vi "SweepCtrlSineCurrent_ver1.0.vi"(7 "Keithley 6221":T1={"Delta "=FALSE, "Const I "=FALSE, "Pulse Delta "=FALSE, "Sine Wave "=FALSE, "From I_HI (A)"=0.0, "From I (A)"=0.0, "I_LO (A)"=0.0, "From I_H (A)"=0.0, "I_L (A)"=0.0, "Freq (Hz)"=13.259, "From I_Sin (A)"=0.0, "DC Offset (A)"=0.0, "Delay Time (s)"=1.0, "Pulse Width (s)"=0.012, "Delay (s)"=0.011966, "To I (A)"=0.0, "ASymmetric?"=FALSE, "To I_HI (A)"=0.0, "To I_H (A)"=0.0, "To I_Sin (A)"=0.0, "GPIB ADR"=0, "Sweep Mode"=0, "Delta Unit"="V", "2182A range (V)"=0.01, "6221 Compliance (V)"=10.0} {"Sweep Mode" items=["Linear", "Log", "Exp", "Inverse", "Manual"]; "GPIB ADR" items=["None"=0, "12"=12, "13"=13]; "To I_Sin (A)" format="%#.5p"; "To I_H (A)" format="%#.5p"; "To I_HI (A)" format="%#.5p"; "To I (A)" format="%#.5p"; "Delay (s)" format="%.3p"; "Pulse Width (s)" format="%.3p"; "Delay Time (s)" format="%#.5p"; "DC Offset (A)" format="%#.5p"; "From I_Sin (A)" format="%#.5p"; "Freq (Hz)" format="%#_6p"; "I_L (A)" format="%#.5p"; "From I_H (A)" format="%#.5p"; "I_LO (A)" format="%#.5p"; "From I (A)" format="%#.5p"; "From I_HI (A)" format="%#.5p"}, 8 "error in (no error)":errorcluster, 9 "Set pt change flag":bool, 10 "DC St. Pt.":dbl, 11 "GPIB ADR":u16) -> (0 "error out":errorcluster)   [LabVIEW 2012]
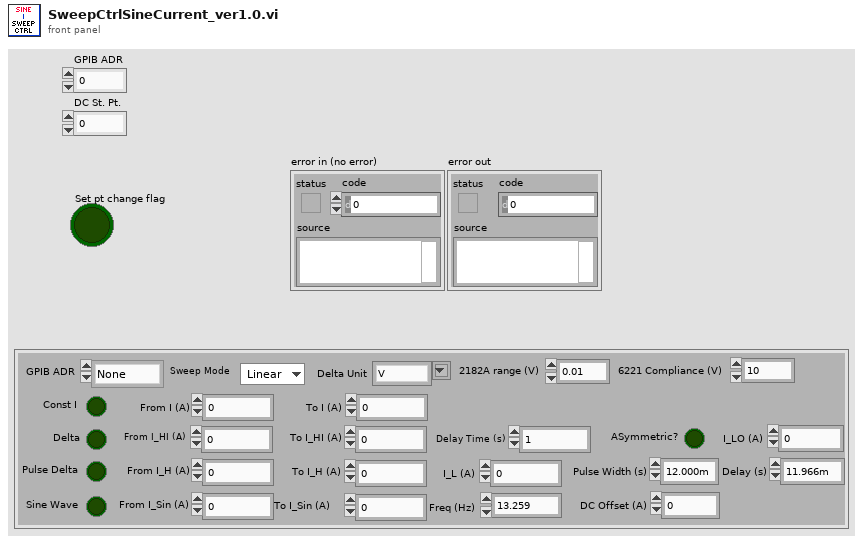
[diagram p1: front panel]
types:
  T1 = cluster{"Delta ":bool, "Const I ":bool, "Pulse Delta ":bool, "Sine Wave ":bool, "From I_HI (A)":dbl, "From I (A)":dbl, "I_LO (A)":dbl, "From I_H (A)":dbl, "I_L (A)":dbl, "Freq (Hz)":dbl, "From I_Sin (A)":dbl, "DC Offset (A)":dbl, "Delay Time (s)":dbl, "Pulse Width (s)":dbl, "Delay (s)":dbl, "To I (A)":dbl, "ASymmetric?":bool, "To I_HI (A)":dbl, "To I_H (A)":dbl, "To I_Sin (A)":dbl, "GPIB ADR":u16, "Sweep Mode":u8, "Delta Unit":string, "2182A range (V)":dbl, "6221 Compliance (V)":dbl}
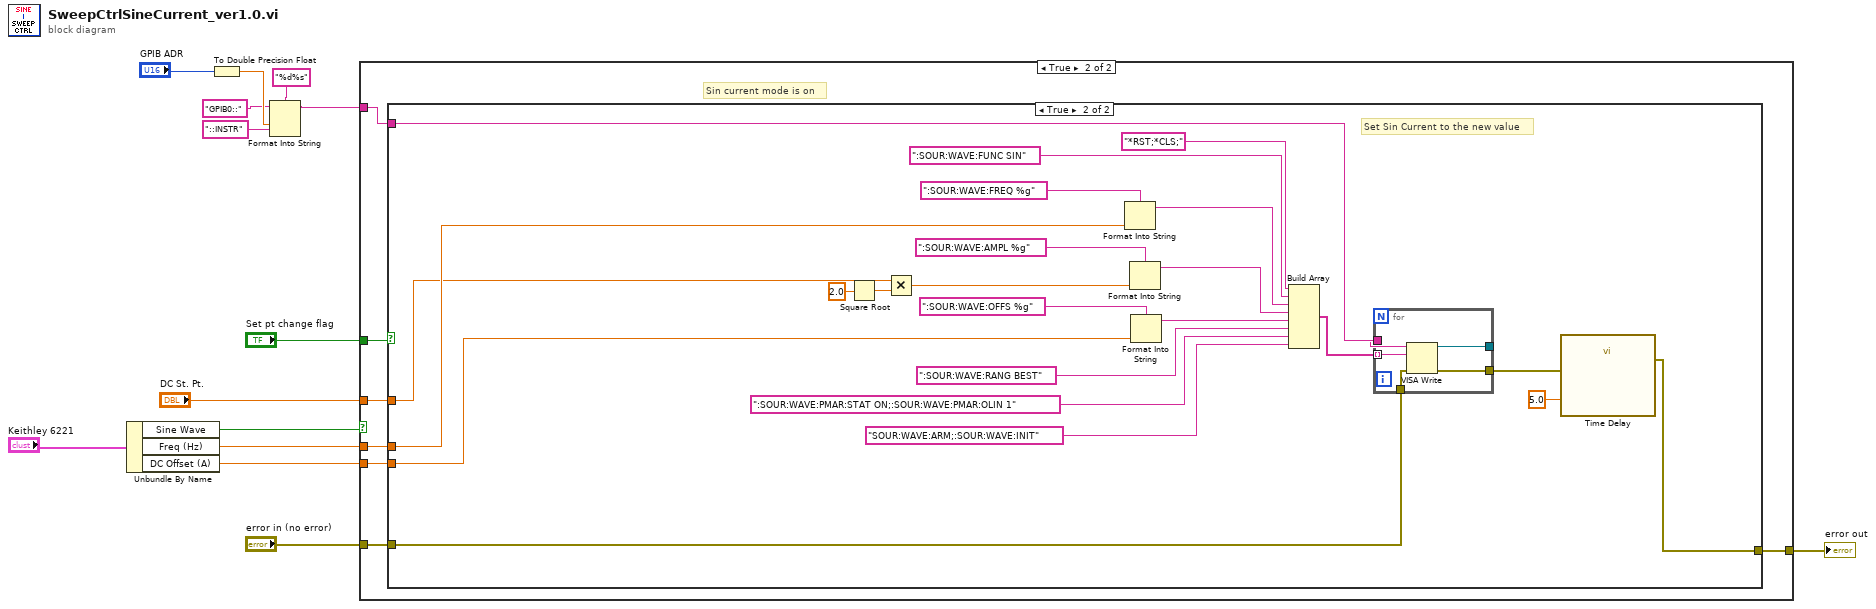
[diagram p0: block diagram]
diagram:
  n1 = Unbundle By Name("Keithley 6221") -> ("Sine Wave"=w9:bool, "Freq (Hz)"=w3:dbl, "DC Offset (A)"=w2:dbl)
  n2 = To Double Precision Float(number="GPIB ADR") -> (double precision float=w13:dbl)
  n3 = Format Into String(format string="%d%s" ("Removes all labels from the string"), initial string="GPIB0::", w13, "::INSTR") -> (resulting string=w8:string)  [unwired: 1 in, 1 out]
  n4 = case shown="True" w9 {
    tunnel: "Set pt change flag" -> [_ w22]
    tunnel: w8 -> [_ w21]
    tunnel: "DC St. Pt." -> [_ w20]
    tunnel: w2 -> [_ w19]
    tunnel: w3 -> [_ w18]
    tunnel: "error in (no error)" -> [w15 w17]
    tunnel: [w15 w16] -> w5
    frame False {
      # "Delta mode is off"
    }
    frame True {
      # "Sin current mode is on"
      n5 = case shown="True" w22 {
        tunnel: w21 -> [_ w46]
        tunnel: w20 -> [_ w35]
        tunnel: w19 -> [_ w32]
        tunnel: w18 -> [_ w39]
        tunnel: w17 -> [w23 w42]
        tunnel: [w23 w24] -> w16
        frame False {
          # "Set Values are not changed"
        }
        frame True {
          # "Set Sin Current to the new value"
          n6 = Square Root(x=2.0 ("y")) -> (sqrt(x)=w37:dbl)
          n7 = Multiply(x=w35, y=w37) -> (x*y=w34:dbl)
          n8 = Format Into String(format string=":SOUR:WAVE:FREQ %g", w39) -> (resulting string=w28:string)  [unwired: 2 in, 1 out]
          n9 = Format Into String(format string=":SOUR:WAVE:AMPL %g", w34) -> (resulting string=w27:string)  [unwired: 2 in, 1 out]
          n10 = Format Into String(format string=":SOUR:WAVE:OFFS %g", w32) -> (resulting string=w44:string)  [unwired: 2 in, 1 out]
          n11 = Build Array("*RST;*CLS;" ("write buffer"), ":SOUR:WAVE:FUNC SIN" ("format string"), w28, w27, w44, ":SOUR:WAVE:RANG BEST" ("format string"), ":SOUR:WAVE:PMAR:STAT ON;:SOUR:WAVE:PMAR:OLIN 1", "SOUR:WAVE:ARM;:SOUR:WAVE:INIT" ("write buffer")) -> (w43:string[])
          n12 = for {
            tunnel: w43 -> [w51] mode=indexing
            tunnel: w46 -> [w50]
            tunnel: [w49] -> w25
            tunnel: w42 -> [w48]
            tunnel: [w47] -> _
            n13 = VISA Write(VISA resource name=w50, write buffer=w51, error in (no error)=w48) -> (VISA resource name out=w47:refnum<visa-resource-name>, error out=w49:errorcluster)  [unwired: 1 out]
          }
          n14 = call "Time Delay"("error in (no error)"=w25, "Delay Time (s)"=5.0) -> ("error out"=w24:errorcluster)  [unwired: 9 in]
        }
      }
    }
  }
  "error out" <- w5
